vi "Get BD Monitor.vi"(8 "error in (no error)":errorcluster, 11 "VI Ref In":refnum<vi>) -> (0 "error out":errorcluster, 2 "Monitor Bounds":T1, 3 "VI Ref Out":refnum<vi>)   [LabVIEW 2019, in "Window.lvlib"]
doc: "Find the bounds of the monitor the specified VI's block diagram is visible on. Bounds are in screen coordinates. If there is an error, returns the primary display bounds."
uses:
  Window.lvlib
  User32.dll
  <vilib>/Utility/miscctls.llb/LVRectTypeDef.ctl
  _2D/2D.lvlib
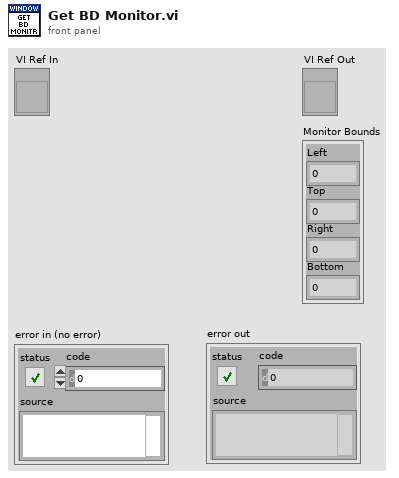
[diagram p1: front panel]
types:
  T1 = typedef "LVRectTypeDef.ctl" = cluster{"Left":i16, "Top":i16, "Right":i16, "Bottom":i16}
  T2 = cluster{"cbSize (DWORD)":u32, "rcMonitor (RECT)":cluster{"left (LONG)":i32, "top (LONG)":i32, "right (LONG)":i32, "bottom (LONG)":i32}, "rcWork (RECT)":cluster{"left (LONG)":i32, "top (LONG)":i32, "right (LONG)":i32, "bottom (LONG)":i32}, "dwFlags (DWORD)":u32}
  T3 = typedef "LVAllMonitorsDisplayTypeDef.ctl" = cluster{"Bounds":cluster{"Left":i16, "Top":i16, "Right":i16, "Bottom":i16}, "Depth":i16}[]
  T4 = cluster{"Left":i16, "Top":i16, "Right":i16, "Bottom":i16}
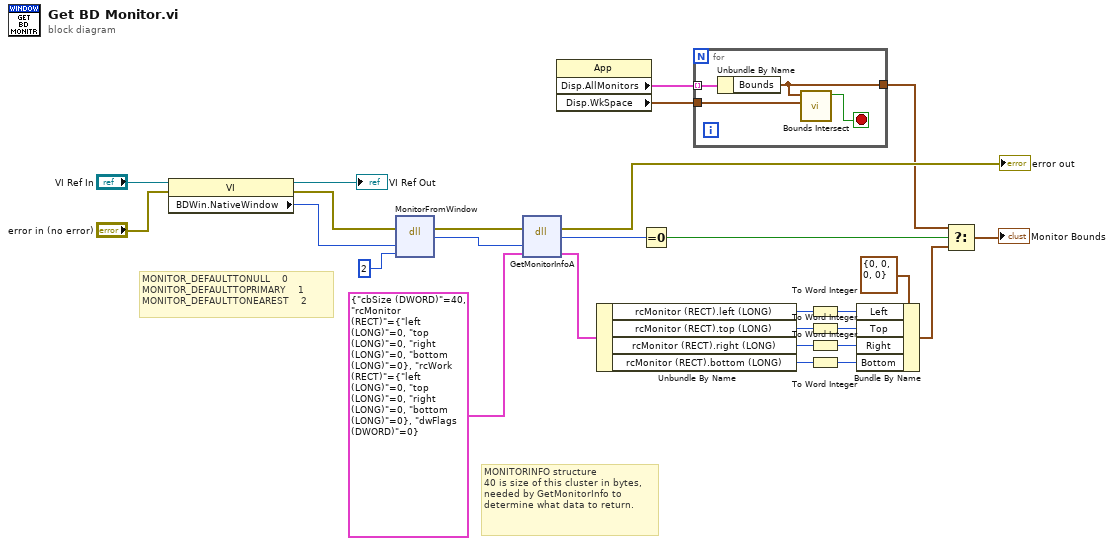
[diagram p0: block diagram]
diagram:
  # "MONITORINFO structure\n40 is size of this cluster in bytes, needed by GetMonitorInfo to determine what data to return."
  # "MONITOR_DEFAULTTONULL    0\nMONITOR_DEFAULTTOPRIMARY    1\nMONITOR_DEFAULTTONEAREST    2"
  n1 = property class="VI"(reference="VI Ref In", error in="error in (no error)") -> (reference out=→"VI Ref Out":refnum<vi>, error out=w24:errorcluster, "BDWin.NativeWindow"=w21:u64)
  n2 = dll-call lib="user32.dll" fn="MonitorFromWindow"(error in=w24, "hWnd"=w21, "dwFlags"=u32 2) -> (error out=w23:errorcluster, "hMonitor"=w26:i32)  [unwired: 3 in, 2 out]
  n3 = dll-call lib="user32.dll" fn="GetMonitorInfoA"(error in=w23, "hMonitor"=w26, "lpmi"=T2 {"cbSize (DWORD)"=40, "rcMonitor (RECT)"={"left (LONG)"=0, "top (LONG)"=0, "right (LONG)"=0, "bottom (LONG)"=0}, "rcWork (RECT)"={"left (LONG)"=0, "top (LONG)"=0, "right (LONG)"=0, "bottom (LONG)"=0}, "dwFlags (DWORD)"=0}) -> (error out=→"error out":errorcluster, "success"=w10:i32, "lpmi"=w19:T2)  [unwired: 3 in, 1 out]
  n4 = property class="App"() -> ("Disp.AllMonitors"=w3:T3, "Disp.WkSpace"=w2:T1)  [unwired: 2 in, 2 out]
  n5 = Unbundle By Name(w19) -> ("rcMonitor (RECT).left (LONG)"=w18:i32, "rcMonitor (RECT).top (LONG)"=w17:i32, "rcMonitor (RECT).right (LONG)"=w16:i32, "rcMonitor (RECT).bottom (LONG)"=w15:i32)
  n6 = Equal To 0?(x=w10) -> (x = 0?=w9:bool)
  n7 = for {
    tunnel: w3 -> [w31] mode=indexing
    tunnel: w2 -> [w30]
    tunnel: [w28] -> w1
    stop <- w29 stop-if-true
    n8 = Unbundle By Name(w31) -> ("Bounds"=w28:T4)
    n9 = call "Bounds Intersect.vi"("Bounds 2"=w30, "Bounds 1"=w28) -> ("Intersect?"=w29:bool)  [unwired: 9 in]
  }
  n10 = To Word Integer(number=w18) -> (16bit integer=w11:i16)
  n11 = To Word Integer(number=w17) -> (16bit integer=w12:i16)
  n12 = To Word Integer(number=w16) -> (16bit integer=w13:i16)
  n13 = To Word Integer(number=w15) -> (16bit integer=w14:i16)
  n14 = Bundle By Name(cluster=T1 {"Left"=0, "Top"=0, "Right"=0, "Bottom"=0} ("Display:Primary Workspace"), "Left"=w11, "Top"=w12, "Right"=w13, "Bottom"=w14) -> (w8:T1)
  n15 = Select(t=w1, s=w9, f=w8) -> (s? t:f=→"Monitor Bounds":T1)
